vi "CODMn启动命令 (子VI).vi"(9 "强制切换":bool, 10 "CODMn量程切换":enum32{"H", "L", "AUTO"}(ring)=enum."AUTO", 11 "启动测量模式":T1) -> ()   [LabVIEW 2016, in "斯坦道CODMn.lvlib"]
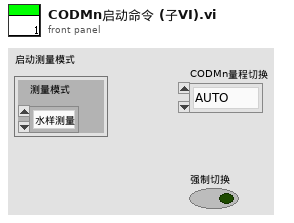
[diagram p1: front panel]
types:
  T1 = cluster{"测量模式":enum16{"水样测量", "标样核查", "零点核查", "跨度核查", "空白测试", "加标回收", "平行样", "校零", "校标"}}
  T2 = cluster{"命令":string, "测量模式":enum16{"水样测量", "标样核查", "零点核查", "跨度核查", "空白测试", "加标回收", "平行样", "校零", "校标"}, "CODMn量程切换":enum32{"H", "L", "AUTO"}}
  T3 = enum16{"水样测量", "标样核查", "零点核查", "跨度核查", "空白测试", "加标回收", "平行样", "校零", "校标"}
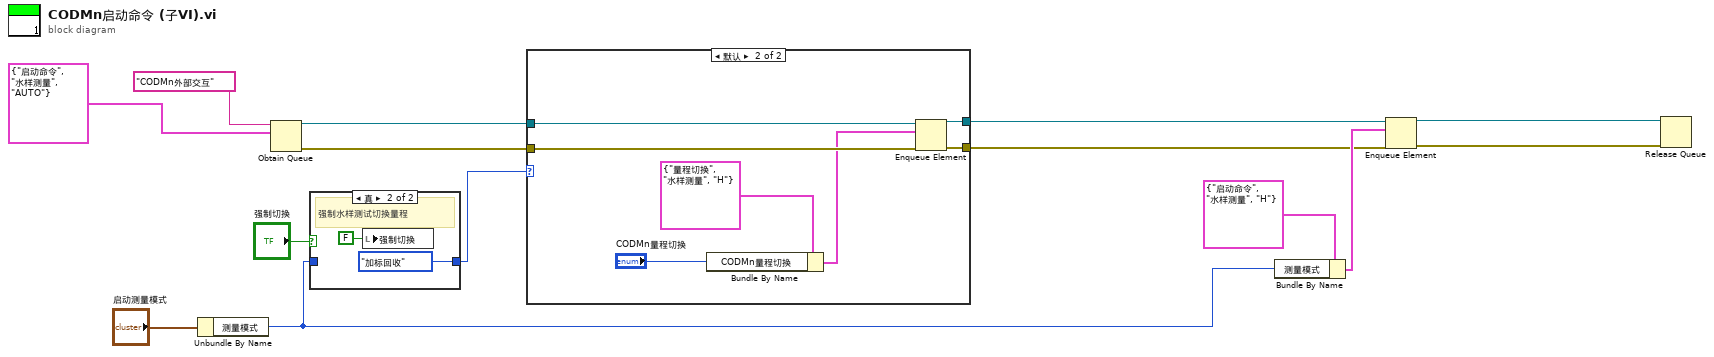
[diagram p0: block diagram]
diagram:
  n1 = Unbundle By Name("启动测量模式") -> ("测量模式"=w2:T3)
  n2 = Obtain Queue(name (unnamed)="CODMn外部交互" ("名称（未命名）"), element data type=T2 {"命令"="启动命令", "测量模式"=enum."水样测量", "CODMn量程切换"=enum."AUTO"} ("元素")) -> (queue out=w7:refnum<queue>, error out=w6:errorcluster)  [unwired: 3 in, 1 out]
  n3 = case shown="真" "强制切换" {
    tunnel: w2 -> [w15 _]
    tunnel: [w15 T3."加标回收" ("测量模式")] -> w1
    frame False {
    }
    frame True {
      # "强制水样测试切换量程"
      n4 = local write "强制切换"(FALSE ("强制切换")) -> ()
    }
  }
  n5 = case shown="默认" w1 {
    tunnel: w7 -> [w19 w26]
    tunnel: w6 -> [w18 w25]
    tunnel: [w19 w24] -> w5
    tunnel: [w18 w23] -> w4
    frame "水样测量" {
    }
    frame Default {
      n6 = Bundle By Name(cluster=T2 {"命令"="量程切换", "测量模式"=enum."水样测量", "CODMn量程切换"=enum."H"} ("元素"), "CODMn量程切换"="CODMn量程切换") -> (w21:T2)
      n7 = Enqueue Element(queue=w26, element=w21, error in (no error)=w25) -> (queue out=w24:refnum<queue>, error out=w23:errorcluster)  [unwired: 1 in, 1 out]
    }
  }
  n8 = Bundle By Name(cluster=T2 {"命令"="启动命令", "测量模式"=enum."水样测量", "CODMn量程切换"=enum."H"} ("元素"), "测量模式"=w2) -> (w8:T2)
  n9 = Enqueue Element(queue=w5, element=w8, error in (no error)=w4) -> (queue out=w12:refnum<queue>, error out=w11:errorcluster)  [unwired: 1 in, 1 out]
  n10 = Release Queue(queue=w12, error in (no error)=w11) -> ()  [unwired: 1 in, 3 out]
